vi "toml_error_syntax.vi"(8 "error in (no error)":errorcluster, 9 "line":i32, 10 "toml":string) -> (0 "error out":errorcluster)   [LabVIEW 2017]
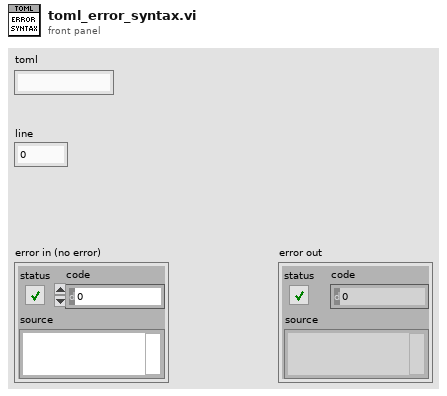
[diagram p1: front panel]
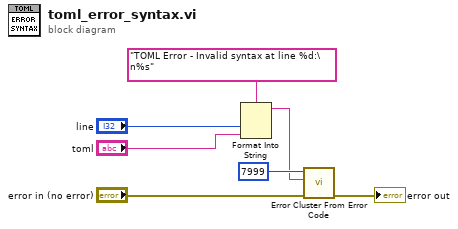
[diagram p0: block diagram]
diagram:
  n1 = Format Into String(format string="TOML Error - Invalid syntax at line %d:\n%s", "line", "toml") -> (resulting string=w3:string)  [unwired: 2 in, 1 out]
  n2 = call <vilib>:"Error Cluster From Error Code.vi"("error in (no error)"="error in (no error)", "error message (\"\")"=w3, "error code (0)"=7999) -> ("error out"=→"error out":errorcluster)  [unwired: 6 in]
